vi "Get pixel X-Y position.vi"(10 "Cell Details Cluster":T1={"Cell Position"=16, "Cell Label"="", "Pixel to measure"=0, "Area (cm^2)"=0.126, "Variable"="", "Variable value"="", "Scan settings in queue"=0, "Light or dark"="", "Measurement Type"=""} {"Pixel to measure" items=["All", "1", "2", "3", "4", "5", "6", "7", "8"]}) -> (0 "Pin":dbl, 2 "Y position":string, 3 "X position":string)   [LabVIEW 2011]
uses:
  <vilib>/Utility/file.llb/Read From Spreadsheet File (DBL).vi
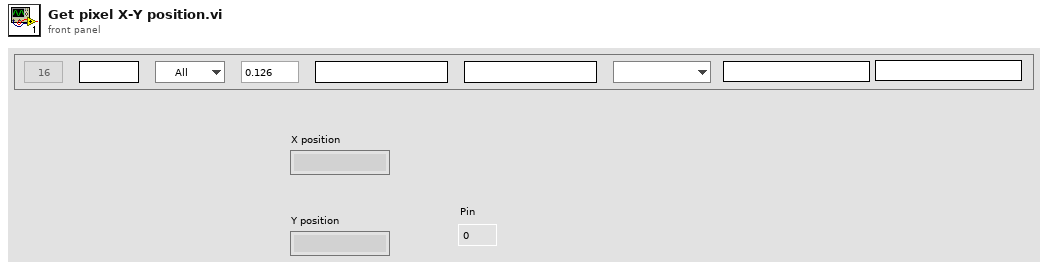
[diagram p1: front panel]
types:
  T1 = cluster{"Cell Position":i32, "Cell Label":string, "Pixel to measure":u16, "Area (cm^2)":dbl, "Variable":string, "Variable value":string, "Scan settings in queue":u16, "Light or dark":string, "Measurement Type":string}
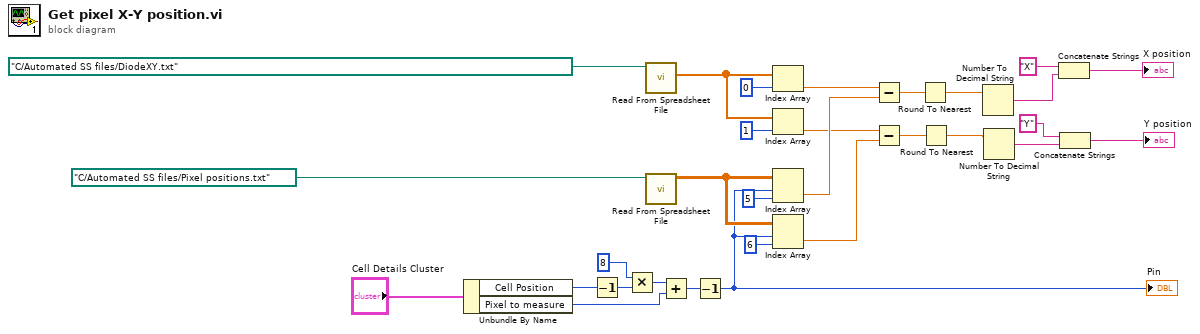
[diagram p0: block diagram]
diagram:
  n1 = Unbundle By Name("Cell Details Cluster") -> ("Cell Position"=w27:i32, "Pixel to measure"=w25:u16)
  n2 = Decrement(x=w27) -> (x-1=w28:i32)
  n3 = Multiply(x=8, y=w28) -> (x*y=w26:i32)
  n4 = call-poly <vilib>:"Read From Spreadsheet File.vi"("file path (dialog if empty)"=path "C:/Automated SS files/DiodeXY.txt") -> ("first row"=w20:dbl[])  [unwired: 6 in, 4 out]
  n5 = call-poly <vilib>:"Read From Spreadsheet File.vi"("file path (dialog if empty)"=path "C:/Automated SS files/Pixel positions.txt") -> ("all rows"=w23:dbl[][])  [unwired: 6 in, 4 out]
  n6 = Add(x=w26, y=w25) -> (x+y=w2:i32)
  n7 = Decrement(x=w2) -> (x-1=w1:i32)
  "Pin" <- w1
  n8 = Index Array(array=w20, index=0) -> (element=w17:dbl)
  n9 = Index Array(array=w20, index=1) -> (element=w15:dbl)
  n10 = Index Array(array=w23, index (row)=w1, index (col)=5) -> (element=w16:dbl)
  n11 = Index Array(array=w23, index (row)=w1, index (col)=6) -> (element=w14:dbl)
  n12 = Subtract(x=w17, y=w16) -> (x-y=w13:dbl)
  n13 = Subtract(x=w15, y=w14) -> (x-y=w12:dbl)
  n14 = Round To Nearest(number=w13) -> (nearest integer value=w11:dbl)
  n15 = Round To Nearest(number=w12) -> (nearest integer value=w10:dbl)
  n16 = Number To Decimal String(number=w11) -> (decimal integer string=w8:string)  [unwired: 1 in]
  n17 = Number To Decimal String(number=w10) -> (decimal integer string=w7:string)  [unwired: 1 in]
  n18 = Concatenate Strings("X", w8) -> (→"X position":string)
  n19 = Concatenate Strings("Y", w7) -> (→"Y position":string)
